vi "Set scan parameters from file.vi"(6 "error in":errorcluster, 9 "Path":path) -> (0 "error out":errorcluster, 2 "bin numbers":cluster{"Bin #s":i32[]}[](array[cluster]), 3 "States Out":string, 4 "first scan cmd":string)   [LabVIEW 2018]
uses:
  <vilib>/Utility/config.llb/NI_LVConfig.lvlib
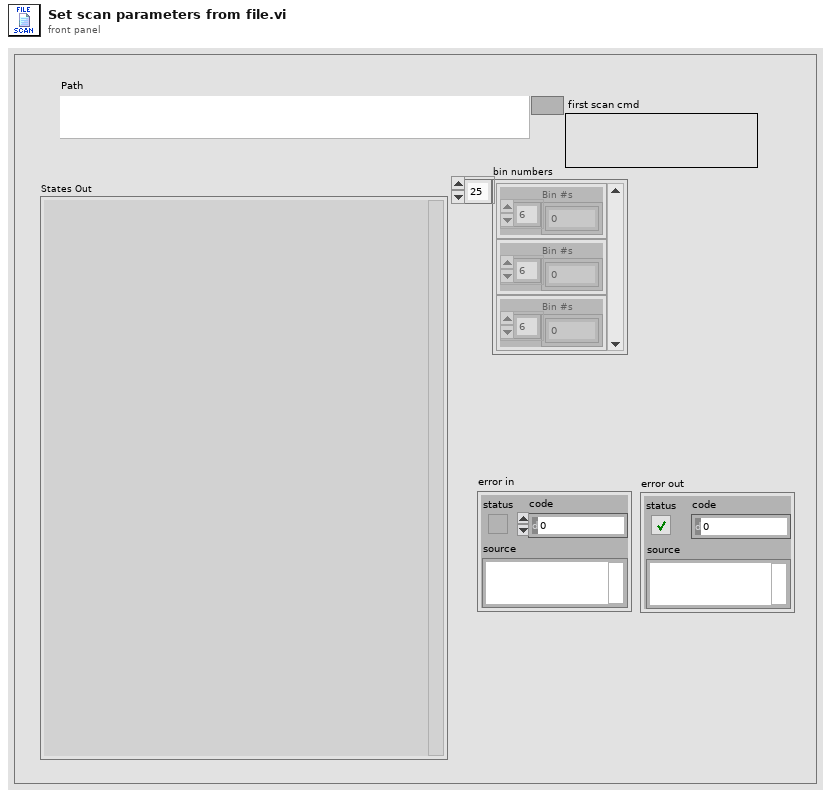
[diagram p1: front panel]
types:
  T1 = typedef "NI_LVConfig.lvlib/Config Data RefNum.ctl" = refnum<k1>
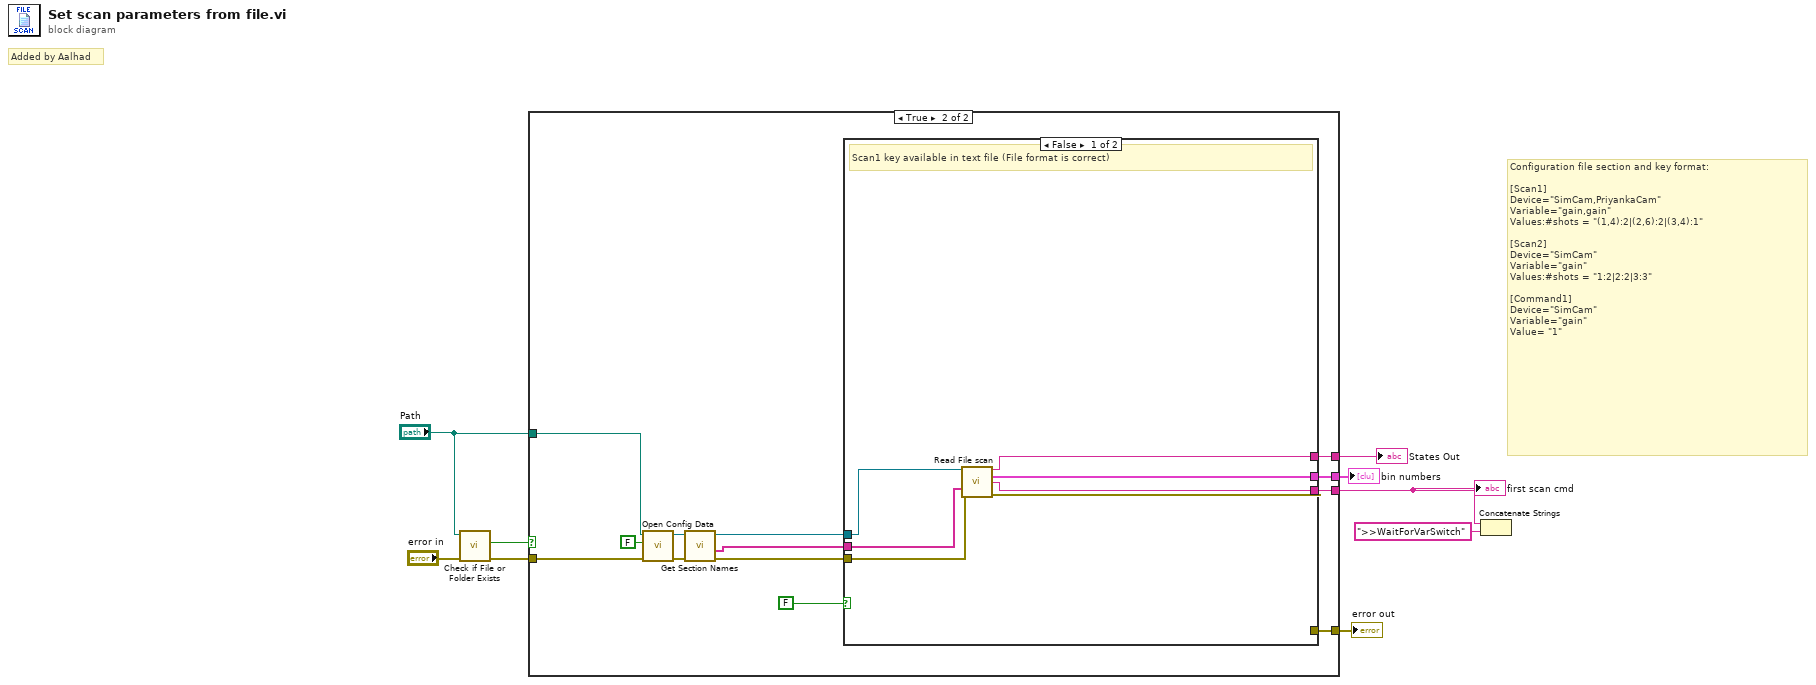
[diagram p0: block diagram]
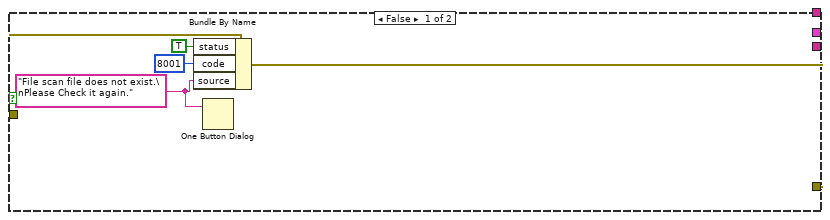
[diagram p2: hidden frame]
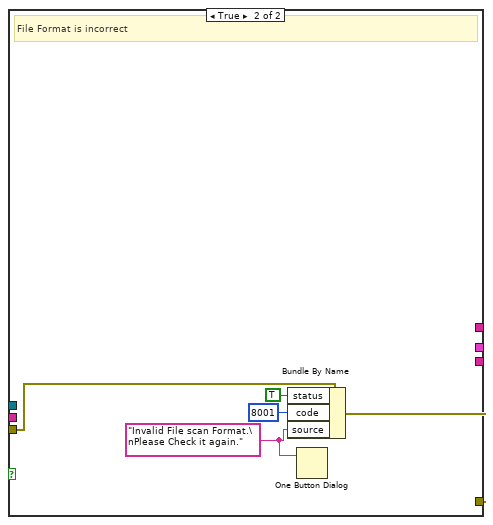
[diagram p3: hidden frame]
diagram:
  # "Configuration file section and key format:\n\n[Scan1]\nDevice=\"SimCam,PriyankaCam\" \nVariable=\"gain,gain\"\nValues:#shots = \"(1,4):2|(2,6):2|(3,4):1\"\n\n[Scan2]\nDevice=\"SimCam\"\nVariable=\"gain\"\nValues:#shots = \"1:2|2:2|3:3\"\n\n[Command1]\nDevice=\"SimCam\" \nVariable=\"gain\"\nValue= \"1\""
  # "Added by Aalhad"
  n1 = call <vilib>:"Check if File or Folder Exists.vi"("error in (no error)"="error in", "path"="Path") -> ("error out"=w6:errorcluster, "file or folder exists?"=w5:bool)  [unwired: 7 in, 1 out]
  n2 = case shown="True" w5 {
    tunnel: [w10 w27] -> w9
    tunnel: "Path" -> [_ w21]
    tunnel: w6 -> [w11 w20]
    tunnel: [_ w17] -> w4
    tunnel: [_ w16] -> w3
    tunnel: [_ w15] -> w2
    frame False {
      w12 = "File scan file does not exist.\nPlease Check it again." ("message")
      n3 = Bundle By Name(cluster=w11, "status"=TRUE, "code"=8001, "source"=w12) -> (w10:errorcluster)
      n4 = One Button Dialog(message=w12) -> ()  [unwired: 1 in, 1 out]
    }
    frame True {
      n5 = call <vilib>:"Open Config Data.vi"("error in (no error)"=w20, "create file if necessary (T)"=FALSE ("create file if necessary? (T)"), "configuration file path"=w21) -> ("error out"=w24:errorcluster, "refnum"=w25:T1)  [unwired: 6 in, 1 out]
      n6 = call <vilib>:"Get Section Names.vi"("error in (no error)"=w24, "refnum"=w25) -> ("error out"=w22:errorcluster, "section names"=w18:string[], "refnum out"=w23:T1)  [unwired: 7 in]
      n7 = case shown="False" FALSE {
        tunnel: w23 -> [w34 _]
        tunnel: w22 -> [w33 w37]
        tunnel: [w32 w36] -> w27
        tunnel: w18 -> [w31 _]
        tunnel: [w30 _] -> w17
        tunnel: [w28 _] -> w16
        tunnel: [w29 _] -> w15
        frame False {
          # "Scan1 key available in text file (File format is correct)"
          n8 = call "Read File scan.vi"("Refnum in"=w34, "section names"=w31, "error in (no error)"=w33) -> ("States Out"=w30:string, "bin numbers"=w28:cluster{"Bin #s":i32[]}[], "first scan cmd"=w29:string, "error out"=w32:errorcluster)  [unwired: 8 in, 1 out]
        }
        frame True {
          w35 = "Invalid File scan Format.\nPlease Check it again." ("message")
          # "File Format is incorrect"
          n9 = Bundle By Name(cluster=w37, "status"=TRUE, "code"=8001, "source"=w35) -> (w36:errorcluster)
          n10 = One Button Dialog(message=w35) -> ()  [unwired: 1 in, 1 out]
        }
      }
    }
  }
  "error out" <- w9
  "States Out" <- w4
  "first scan cmd" <- w2
  "bin numbers" <- w3
  n11 = Concatenate Strings(w2, ">>WaitForVarSwitch" ("string")) -> ()  [unwired: 1 out]
